vi "to_data.vi"(11 "Bytes in":refnum<class "Bytes.lvclass">) -> (3 "byte array":u8[](array[numeric]))   [LabVIEW 2020, in "variant.lvlib" / "Bytes.lvclass"]
uses:
  Bytes.lvclass
  Bytes.lvclass/Bytes.ctl
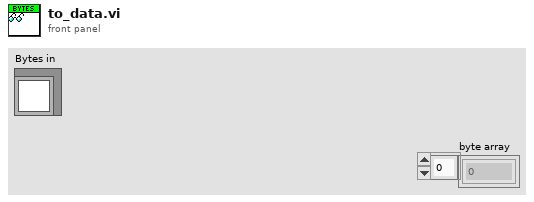
[diagram p1: front panel]
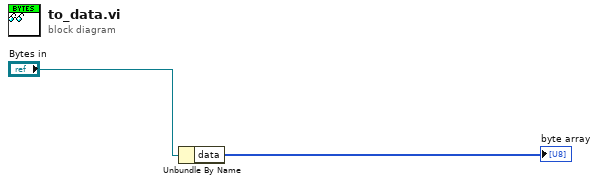
[diagram p0: block diagram]
diagram:
  n1 = Unbundle By Name("Bytes in") -> ("data"=→"byte array":u8[])
